vi "close.vi"(8 "error in (no error)":errorcluster, 11 "Counter in":refnum<class "Counter.lvclass">) -> (0 "error out":errorcluster, 3 "Counter out":refnum<class "Counter.lvclass">)   [LabVIEW 2014, in "Counter.lvclass"]
uses:
  Counter.lvclass
  Counter.lvclass/Counter.ctl
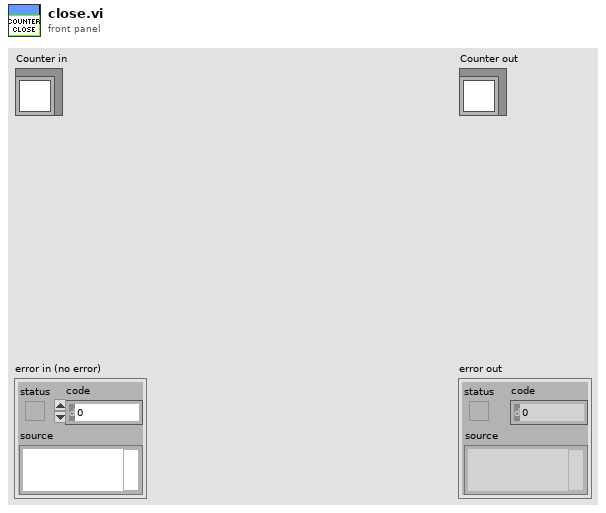
[diagram p1: front panel]
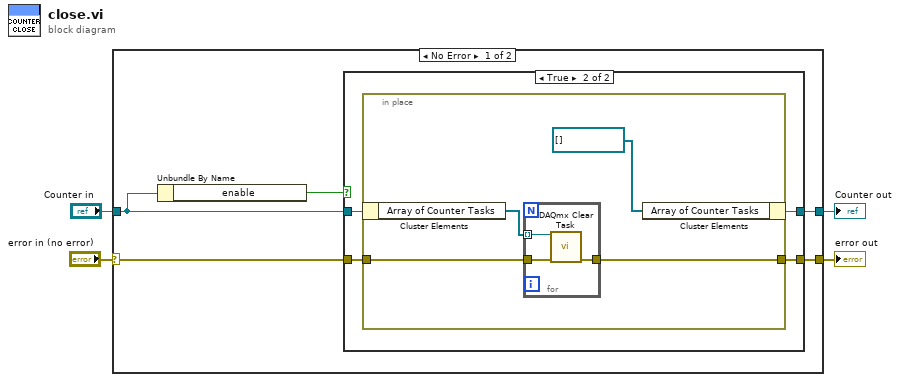
[diagram p0: block diagram]
diagram:
  n1 = case shown="No Error" "error in (no error)" {
    selector: "error in (no error)" -> [w8 w24]
    tunnel: [w7 w24] -> w3
    tunnel: [w5 w23] -> w1
    tunnel: "Counter in" -> [w6 w23]
    frame No Error {
      n2 = Unbundle By Name(w6) -> ("enable"=w9:bool)
      n3 = case shown="True" w9 {
        tunnel: w8 -> [w11 w15]
        tunnel: [w11 w14] -> w7
        tunnel: w6 -> [w10 w13]
        tunnel: [w10 w12] -> w5
        frame False {
        }
        frame True {
          n4 = in-place {
            in-place-border: w15 -> [w19]
            in-place-border: [w18] -> w14
            n5 = in-place-cluster #1(w13) -> ("Array of Counter Tasks"=w17:refnum<k21>[])
            n6 = for {
              tunnel: w17 -> [w20] mode=indexing
              tunnel: w19 -> [w22]
              tunnel: [w21] -> w18
              n7 = call <vilib>:"DAQmx Clear Task.vi"("task in"=w20, "error in"=w22) -> ("error out"=w21:errorcluster)  [unwired: 13 out]
            }
            n8 = in-place-cluster #1("Array of Counter Tasks"=refnum<k21>[] []) -> (w12:refnum<class "Counter.lvclass">)
          }
        }
      }
    }
    frame Error {
    }
  }
  "error out" <- w3
  "Counter out" <- w1
